vi "SCPI - Lookup AI Channel Code.vi"(10 "Analog Input Channel Number":i32) -> (2 "Channel Code":i32)   [LabVIEW 2021]
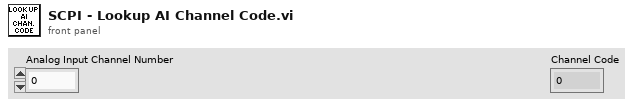
[diagram p1: front panel]
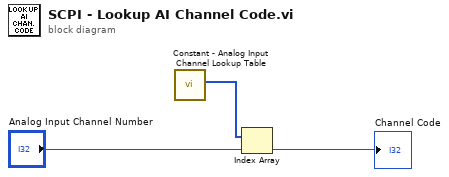
[diagram p0: block diagram]
diagram:
  n1 = call "Constant - Analog Input Channel Lookup Table.vi"() -> ("Analog Channel Lookup Table"=w3:i32[])  [unwired: 11 in]
  n2 = Index Array(array=w3, index="Analog Input Channel Number") -> (element=→"Channel Code":i32)
